vi "Round to Near X.vi"(10 "x":dbl, 11 "input":dbl) -> (2 "round to X":dbl)   [LabVIEW 2018]
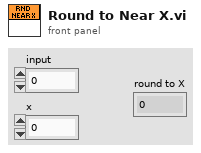
[diagram p1: front panel]
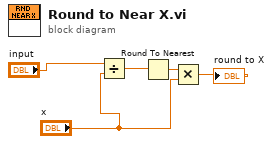
[diagram p0: block diagram]
diagram:
  n1 = Divide(x="input", y="x") -> (x/y=w2:dbl)
  n2 = Round To Nearest(number=w2) -> (nearest integer value=w5:dbl)
  n3 = Multiply(x=w5, y="x") -> (x*y=→"round to X":dbl)
